vi "lab4.vi"() -> ()   [LabVIEW 2017]
panel:
  in  "Display History":bool
  in  "Size of Rectangle":i16
  in  "Send Button":bool
  in  "DAC 2":dbl
  in  "DAC1":dbl
  out "Rec Extra3":dbl
  out "Y":dbl
  out "X":dbl
  in  "stop":bool
  out "2D Picture":picture
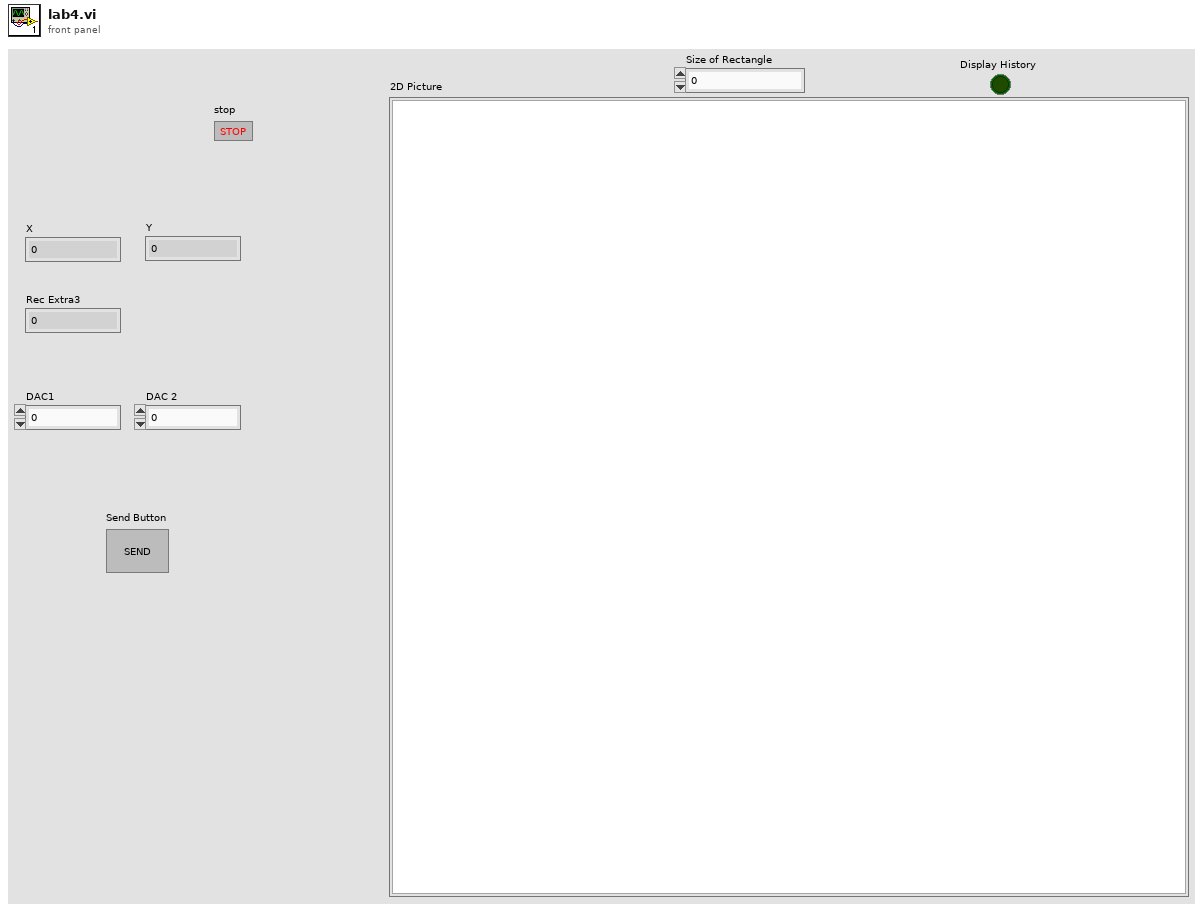
[diagram p1: front panel]
types:
  T1 = enum16{"Standard", "Buffered", "CRLF", "Immediate"}
  T2 = cluster{"Width":u16, "Style":enum32{"Solid", "Dash", "Dot", "DashDot", "DashDotDot"}}
  T3 = cluster{"default value 6":dbl, "default value 7":dbl}
  T4 = cluster{"default value 8":dbl, "default value 9":dbl}
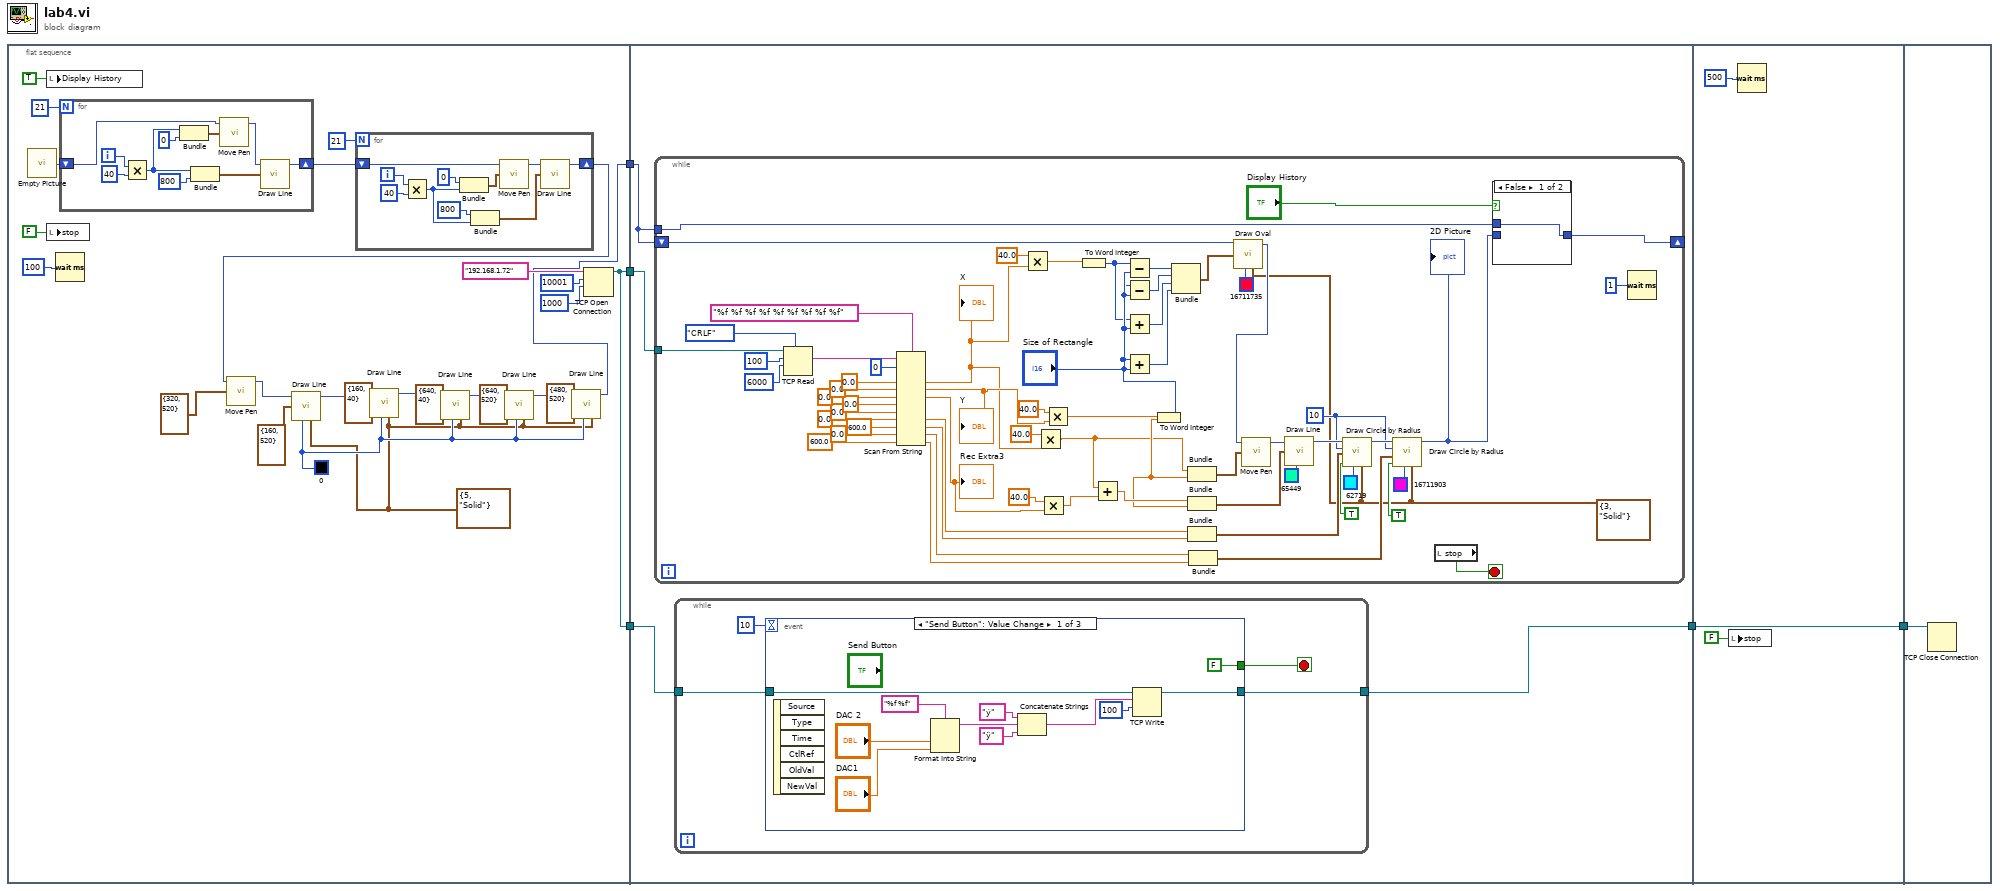
[diagram p0: block diagram]
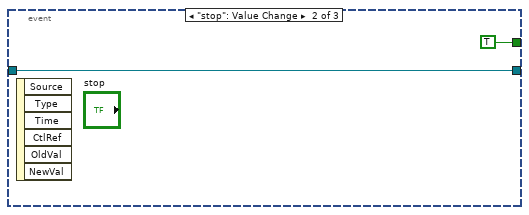
[diagram p3: hidden frame]
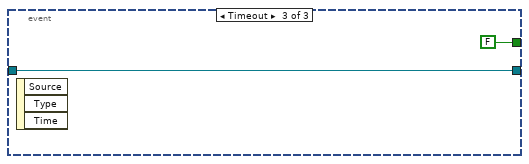
[diagram p4: hidden frame]
diagram:
  n1 = flat-sequence {
    tunnel: [w25] -> w5
    tunnel: [w25] -> w2
    tunnel: [w7] -> w1
    tunnel: w5 -> [w55]
    tunnel: [w54] -> w3
    tunnel: w2 -> [w53]
    tunnel: w1 -> [w52]
    tunnel: [w140] -> w4
    tunnel: w3 -> [w140]
    tunnel: w4 -> [w143]
    frame #0 {
      w13 = u32 0 ("color(black)")
      w6 = T2 {"Width"=5, "Style"=enum."Solid"} ("pen")
      n2 = call "Empty Picture"() -> ("empty picture"=w23:picture)
      n3 = local write "Display History"(TRUE ("Display History")) -> ()
      n4 = local write "stop"(FALSE ("stop")) -> ()
      n5 = Wait (ms)(milliseconds to wait=u32 100) -> ()  [unwired: 1 out]
      n6 = for {
        N: 21 -> [_]
        shift-right: [w49] -> w21
        shift-left: w23 -> [w50]
        i -> [w42]
        n7 = Multiply(x=w42, y=i16 40 ("x 2")) -> (x*y=w43:i32)
        n8 = Bundle(w43, 0) -> (w46:cluster{i32, i32})  [unwired: 1 in]
        n9 = Bundle(w43, 800) -> (w44:cluster{i32, i32})  [unwired: 1 in]
        n10 = call <vilib>:"Move Pen.vi"("new position"=w46, "picture"=w50) -> ("new picture"=w51:picture)  [unwired: 3 in]
        n11 = call <vilib>:"Draw Line.vi"("picture"=w51, "end point"=w44) -> ("new picture"=w49:picture)  [unwired: 7 in]
      }
      n12 = for {
        N: 21 -> [_]
        shift-right: [w39] -> w8
        shift-left: w21 -> [w40]
        i -> [w35]
        n13 = Multiply(x=w35, y=i16 40 ("x 2")) -> (x*y=w32:i32)
        n14 = Bundle(0, w32) -> (w37:cluster{i32, i32})  [unwired: 1 in]
        n15 = Bundle(800, w32) -> (w36:cluster{i32, i32})  [unwired: 1 in]
        n16 = call <vilib>:"Move Pen.vi"("new position"=w37, "picture"=w40) -> ("new picture"=w41:picture)  [unwired: 3 in]
        n17 = call <vilib>:"Draw Line.vi"("picture"=w41, "end point"=w36) -> ("new picture"=w39:picture)  [unwired: 7 in]
      }
      n18 = call <vilib>:"Move Pen.vi"("new position"=cluster{"x":i16, "y":i16} {"x"=320, "y"=520}, "picture"=w8) -> ("new picture"=w19:picture)  [unwired: 3 in]
      n19 = call <vilib>:"Draw Line.vi"("picture"=w19, "end point"=cluster{"x":i16, "y":i16} {"x"=160, "y"=520}, "color(black)"=w13, "pen"=w6) -> ("new picture"=w17:picture)  [unwired: 5 in]
      n20 = call <vilib>:"Draw Line.vi"("picture"=w17, "end point"=cluster{"x":i16, "y":i16} {"x"=160, "y"=40}, "color(black)"=w13, "pen"=w6) -> ("new picture"=w16:picture)  [unwired: 5 in]
      n21 = call <vilib>:"Draw Line.vi"("picture"=w16, "end point"=cluster{"x":i16, "y":i16} {"x"=640, "y"=40}, "color(black)"=w13, "pen"=w6) -> ("new picture"=w15:picture)  [unwired: 5 in]
      n22 = call <vilib>:"Draw Line.vi"("picture"=w15, "end point"=cluster{"x":i16, "y":i16} {"x"=640, "y"=520}, "color(black)"=w13, "pen"=w6) -> ("new picture"=w14:picture)  [unwired: 5 in]
      n23 = call <vilib>:"Draw Line.vi"("picture"=w14, "end point"=cluster{"x":i16, "y":i16} {"x"=480, "y"=520}, "color(black)"=w13, "pen"=w6) -> ("new picture"=w7:picture)  [unwired: 5 in]
      n24 = TCP Open Connection(address="192.168.1.72", remote port or service name=u16 10001, timeout ms (60000)=1000) -> (connection ID=w25:refnum<k5>)  [unwired: 2 in, 1 out]
    }
    frame #1 {
      n25 = while {
        tunnel: w53 -> [w118]
        shift-right: [w97] -> _
        shift-left: w52 -> [w95]
        tunnel: w52 -> [w96]
        stop <- w98 stop-if-true
        w62 = i16 10 ("radius")
        w56 = T2 {"Width"=3, "Style"=enum."Solid"} ("pen")
        n26 = TCP Read(connection ID=w118, bytes to read=100, 7:T1."CRLF" ("mode (standard)"), 9:6000 ("timeout ms (25000)")) -> (data out=w114:string)  [unwired: 1 in, 2 out]
        n27 = Scan From String(format string="%f %f %f %f %f %f %f %f %f", input string=w114, initial scan location=u32 0, default 1=0.0 ("default value 1"), default 2=0.0 ("default value 2"), default 3=0.0 ("default value 3"), default 4=0.0 ("default value 4"), default 5=0.0 ("default value 5"), default 6=0.0 ("default value 6"), default 7=600.0 ("default value 7"), default 8=0.0 ("default value 8"), default 9=600.0 ("default value 9")) -> (output 1=w78:dbl, output 2=w79:dbl, output 3=w86:dbl, output 6=w68:dbl, output 7=w67:dbl, output 8=w60:dbl, output 9=w59:dbl)  [unwired: 3 in, 3 out]
        "Rec Extra3" <- w86
        "Y" <- w79
        "X" <- w78
        n28 = Multiply(x=40.0, y=w78) -> (x*y=w80:dbl)
        n29 = Multiply(x=40.0, y=w78) -> (x*y=w81:dbl)
        n30 = Multiply(x=40.0, y=w86) -> (x*y=w87:dbl)
        n31 = Multiply(x=40.0, y=w79) -> (x*y=w82:dbl)
        n32 = To Word Integer(number=w80) -> (16bit integer=w104:i16)
        n33 = Add(x=w81, y=w87) -> (x+y=w90:dbl)
        n34 = Subtract(x=w104, y="Size of Rectangle") -> (x-y=w103:i16)
        n35 = Add(x=w104, y="Size of Rectangle") -> (x+y=w101:i16)
        n36 = To Word Integer(number=w82) -> (16bit integer=w83:i16)
        n37 = Subtract(x=w83, y="Size of Rectangle") -> (x-y=w102:i16)
        n38 = Add(x=w83, y="Size of Rectangle") -> (x+y=w100:i16)
        n39 = Bundle(w103, w102, w101, w100) -> (w72:cluster{i16, i16, i16, i16})  [unwired: 1 in]
        n40 = Bundle(w81, w82) -> (w91:cluster{dbl, dbl})  [unwired: 1 in]
        n41 = Bundle(w90, w82) -> (w89:cluster{dbl, dbl})  [unwired: 1 in]
        n42 = Bundle("default value 6"=w68, "default value 7"=w67) -> (w66:T3)  [unwired: 1 in]
        n43 = Bundle("default value 8"=w60, "default value 9"=w59) -> (w61:T4)  [unwired: 1 in]
        n44 = call <vilib>:"Draw Oval.vi"("picture"=w95, "rect"=w72, "color(black)"=u32 16711735, "pen"=w56) -> ("new picture"=w92:picture)  [unwired: 5 in]
        n45 = call <vilib>:"Move Pen.vi"("new position"=w91, "picture"=w92) -> ("new picture"=w93:picture)  [unwired: 3 in]
        n46 = call <vilib>:"Draw Line.vi"("picture"=w93, "end point"=w89, "color(black)"=u32 65449) -> ("new picture"=w71:picture)  [unwired: 6 in]
        n47 = call <vilib>:"Draw Circle by Radius.vi"("pen"=w56, "color(black)"=u32 62719, "fill?(F)"=TRUE, "pixel center"=w66, "radius"=w62, "picture"=w71) -> ("new picture"=w64:picture)  [unwired: 5 in]
        n48 = call <vilib>:"Draw Circle by Radius.vi"("pen"=w56, "color(black)"=u32 16711903, "fill?(F)"=TRUE, "pixel center"=w61, "radius"=w62, "picture"=w64) -> ("new picture"=w65:picture)  [unwired: 5 in]
        "2D Picture" <- w65
        n49 = local read "stop"() -> (w98:bool)
        n50 = case shown="False" "Display History" {
          tunnel: w65 -> [_ w120]
          tunnel: [w119 w120] -> w97
          tunnel: w96 -> [w119 _]
          frame False {
          }
          frame True {
          }
        }
        n51 = Wait (ms)(milliseconds to wait=u32 1) -> ()  [unwired: 1 out]
      }
      n52 = while {
        tunnel: w55 -> [w123]
        tunnel: [w122] -> w54
        stop <- w121 stop-if-true
        n53 = event shown="[0] \"Send Button\": Value Change" {
          selector: _ -> [_ _ _]
          dyn-events: _ -> [_ _ _]
          timeout: 10 -> [_ _ _]
          tunnel: w123 -> [w127 w137 w139]
          tunnel: [w126 w137 w139] -> w122
          tunnel: [FALSE TRUE ("stop") FALSE] -> w121
          event "Send Button": Value Change {
            n54 = event-data() -> ()  [unwired: 1 in, 6 out]
            n55 = Format Into String(format string="%f %f", "DAC 2", "DAC1") -> (resulting string=w132:string)  [unwired: 2 in, 1 out]
            n56 = Concatenate Strings("ý" ("string"), w132, "ÿ" ("string")) -> (w129:string)
            n57 = TCP Write(connection ID=w127, data in=w129, 9:100 ("timeout ms (25000)")) -> (connection ID out=w126:refnum<k5>)  [unwired: 1 in, 2 out]
          }
          event "stop": Value Change {
            n58 = event-data() -> ()  [unwired: 1 in, 6 out]
          }
          event Timeout {
            n59 = event-data() -> ()  [unwired: 1 in, 3 out]
          }
        }
      }
    }
    frame #2 {
      n60 = local write "stop"(FALSE ("stop")) -> ()
      n61 = Wait (ms)(milliseconds to wait=u32 500) -> ()  [unwired: 1 out]
    }
    frame #3 {
      n62 = TCP Close Connection(connection ID=w143) -> ()  [unwired: 2 in, 2 out]
    }
  }
